vi "Counter.vi"(8 "error in (no error)":errorcluster, 10 "Units":u16, 11 "SPARC4_AC in":refnum<class "S4GUI.lvclass">) -> (0 "error out":errorcluster, 2 "data out":string, 3 "SPARC4_AC out":refnum<class "S4GUI.lvclass">)   [LabVIEW 2018, in "S4GUI.lvclass"]
uses:
  S4GUI.lvclass
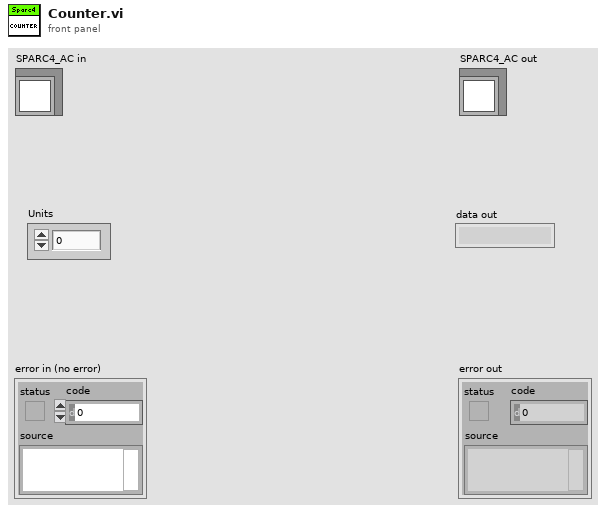
[diagram p1: front panel]
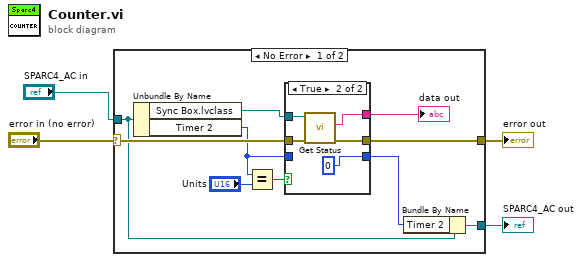
[diagram p0: block diagram]
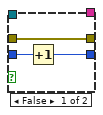
[diagram p2: hidden frame]
diagram:
  n1 = case shown="No Error" "error in (no error)" {
    selector: "error in (no error)" -> [w11 w24]
    tunnel: [w10 w24] -> w3
    tunnel: [w6 w23] -> w1
    tunnel: "SPARC4_AC in" -> [w9 w23]
    frame No Error {
      n2 = Unbundle By Name(w9) -> ("Sync Box.lvclass"=w12:refnum<class "Sync Box.lvclass">, "Timer 2"=w8:u16)
      n3 = Equal?(x=w8, y="Units") -> (x = y?=w13:bool)
      n4 = case shown="True" w13 {
        tunnel: w12 -> [_ w22]
        tunnel: w11 -> [w15 w21]
        tunnel: [w15 w20] -> w10
        tunnel: w8 -> [w17 _]
        tunnel: [w16 u16 0] -> w7
        tunnel: [_ w18] -> w5
        frame False {
          n5 = Increment(x=w17) -> (x+1=w16:u16)
        }
        frame True {
          n6 = call "Get Status.vi"("error in (no error)"=w21, "Sync Box in"=w22) -> ("error out"=w20:errorcluster, "data out"=w18:string)  [unwired: 7 in, 1 out]
        }
      }
      "data out" <- w5
      n7 = Bundle By Name(cluster=w9, "Timer 2"=w7) -> (w6:refnum<class "S4GUI.lvclass">)
    }
    frame Error {
    }
  }
  "error out" <- w3
  "SPARC4_AC out" <- w1
